vi "Stop.vi"(8 "error in (no error)":errorcluster, 11 "Exit in":refnum<class "Exit.lvclass">) -> (0 "error out":errorcluster, 2 "Stop":bool, 3 "Exit out":refnum<class "Exit.lvclass">)   [LabVIEW 2020, in "Exit.lvclass"]
uses:
  Exit.lvclass
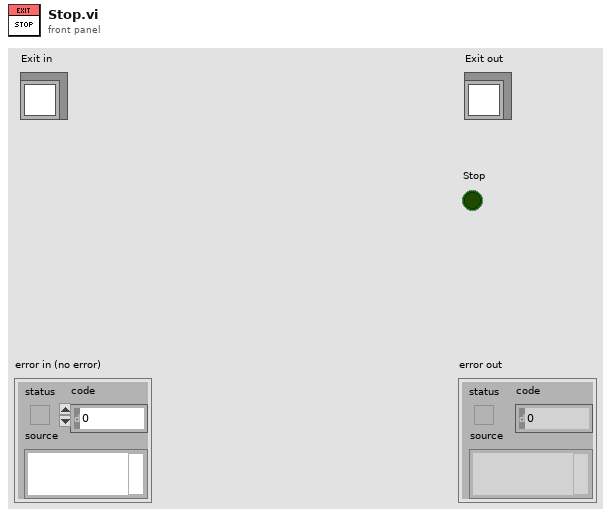
[diagram p1: front panel]
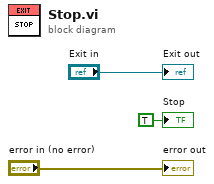
[diagram p0: block diagram]
diagram:
  "error out" <- "error in (no error)"
  "Exit out" <- "Exit in"
  "Stop" <- TRUE ("Stop")
